vi "Configure.vi"(8 "error in (no error)":errorcluster, 11 "Stage_MadCityLab in":refnum<class "Stage_MadCityLab.lvclass">) -> (0 "error out":errorcluster, 3 "Stage_MadCityLab out":refnum<class "Stage_MadCityLab.lvclass">)   [LabVIEW 2020, in "Stage_MadCityLab.lvlib" / "Stage_MadCityLab.lvclass"]
uses:
  Stage_MadCityLab.lvclass
  HAL Layer/Stage/Stage/Stage.lvclass
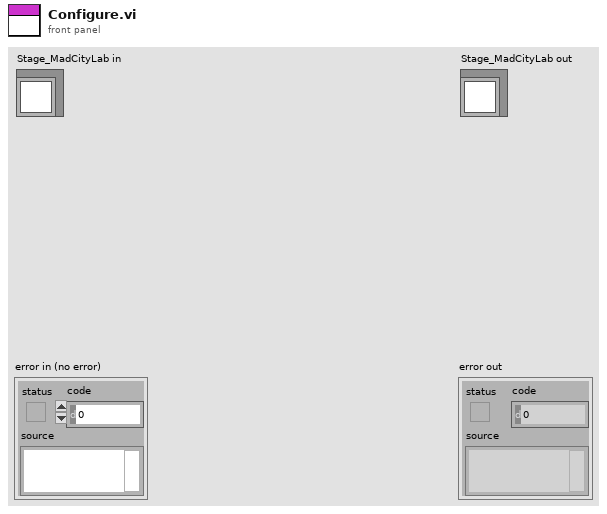
[diagram p1: front panel]
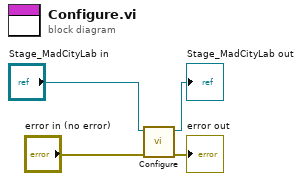
[diagram p0: block diagram]
diagram:
  n1 = call-parent "Configure.vi"("error in (no error)"="error in (no error)", "Device in"="Stage_MadCityLab in") -> ("error out"=→"error out":errorcluster, "Device out"=→"Stage_MadCityLab out":refnum<class "Stage_MadCityLab.lvclass">)  [unwired: 8 in]
